vi "Last Ack.vi"(9 "Error":errorcluster, 10 "Actor":refnum<class "Actor.lvclass">, 11 "Self Actor in":refnum<class "Self Actor.lvclass">) -> (0 "error out":errorcluster, 3 "Self Actor out":refnum<class "Self Actor.lvclass">)   [LabVIEW 2021, in "AAM.lvlib" / "Self Actor.lvclass"]
uses:
  Self Actor.lvclass
  Actor/Actor.lvclass
  Self Actor.lvclass/Self Actor.ctl
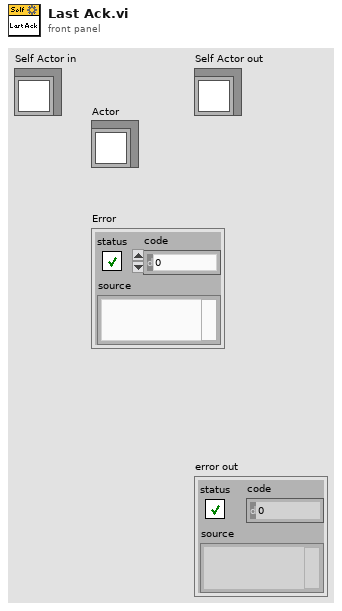
[diagram p1: front panel]
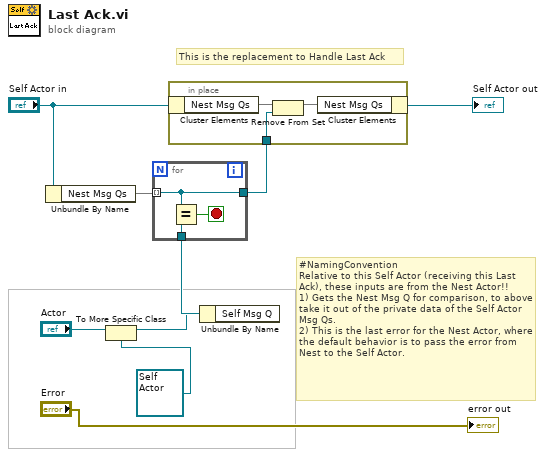
[diagram p0: block diagram]
diagram:
  # "#NamingConvention\nRelative to this Self Actor (receiving this Last Ack), these inputs are from the Nest Actor!! \n1) Gets the Nest Msg Q for comparison, to above take it out of the private data of the Self Actor Msg Qs.\n2) This is the last error for the Nest Actor, where the default behavior is to pass the error from Nest to the Self Actor."
  # "This is the replacement to Handle Last Ack"
  n1 = Unbundle By Name("Self Actor in") -> ("Nest Msg Qs"=w7:set{refnum<class "Msg Q.lvclass">})
  n2 = To More Specific Class(target class=refnum<class "Self Actor.lvclass"> refnum ("Artifex Actor Model.lvlib:Self Actor.lvclass"), reference="Actor") -> (specific class reference=w2:refnum<class "Self Actor.lvclass">)  [unwired: 1 in, 1 out]
  n3 = Unbundle By Name(w2) -> ("Self Msg Q"=w6:refnum<class "Msg Q.lvclass">)
  n4 = for {
    tunnel: w6 -> [w12]
    tunnel: w7 -> [w10] mode=indexing
    tunnel: [w10] -> w5
    stop <- w11 stop-if-true
    n5 = Equal?(x=w10, y=w12) -> (x = y?=w11:bool)
  }
  n6 = in-place {
    in-place-border: w5 -> [w13]
    n7 = in-place-cluster #1("Self Actor in") -> ("Nest Msg Qs"=w14:set{refnum<class "Msg Q.lvclass">})
    n8 = Remove From Set(10:w13, 11:w14) -> (3:w15:set{refnum<class "Msg Q.lvclass">})  [unwired: 1 out]
    n9 = in-place-cluster #1("Nest Msg Qs"=w15) -> (→"Self Actor out":refnum<class "Self Actor.lvclass">)
  }
  "error out" <- "Error"
